vi "Execute.vi"(6 "Index [-1]":i32=-1, 7 "Composite Object":refnum<class "CConfig Object.lvclass">, 8 "error in (no error)":errorcluster, 9 "Results":string[][](array[string]), 11 "Config Query in":refnum<class "If Query.lvclass">) -> (0 "error out":errorcluster, 1 "Results":string[][](array[string]), 2 "Result":bool, 3 "Config Query out":refnum<class "If Query.lvclass">, 4 "Index":i32, 5 "Composite Object":refnum<class "CConfig Object.lvclass">)   [LabVIEW 2013, in "If Query.lvclass"]
doc: "Copyright 2018, Carya Automatisering, Wiebe Walstra."
uses:
  If Query.lvclass
  CConfig Object.lvclass
  If Query.lvclass/If Query.ctl
  CConfig Query.lvclass
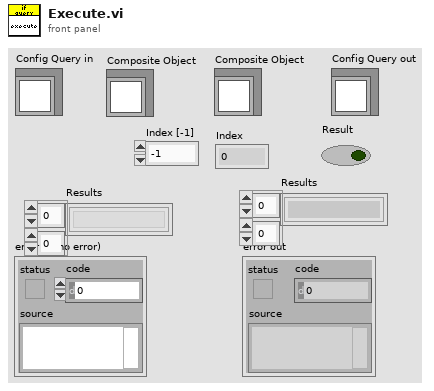
[diagram p1: front panel]
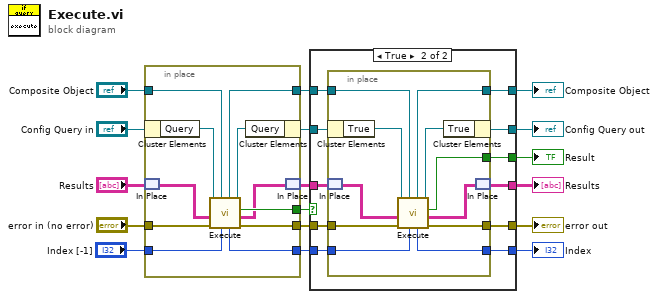
[diagram p0: block diagram]
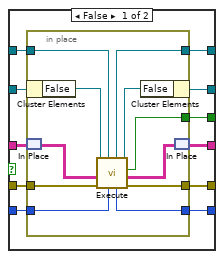
[diagram p2: hidden frame]
diagram:
  n1 = in-place {
    in-place-border: "error in (no error)" -> [w28]
    in-place-border: [w27] -> w15
    in-place-border: [w26] -> w13
    in-place-border: "Composite Object" -> [w25]
    in-place-border: "Index [-1]" -> [w24]
    in-place-border: [w23] -> w5
    in-place-border: [w20] -> w4
    n2 = in-place-cluster #1("Config Query in") -> ("Query"=w22:refnum<class "CConfig Query.lvclass">)
    n3 = in-place-match #2("Results") -> (w19:string[][])
    n4 = call-dynamic "Execute.vi"("Index [-1]"=w24, "Composite Object"=w25, "error in (no error)"=w28, "Results"=w19, "Config Query in"=w22) -> ("error out"=w27:errorcluster, "Results"=w18:string[][], "Result"=w20:bool, "Config Query out"=w21:refnum<class "CConfig Query.lvclass">, "Index"=w23:i32, "Composite Object"=w26:refnum<class "CConfig Object.lvclass">)  [unwired: 1 in]
    n5 = in-place-cluster #1("Query"=w21) -> (w6:refnum<class "If Query.lvclass">)
    n6 = in-place-match #2(w18) -> (w1:string[][])
  }
  n7 = case shown="True" w4 {
    tunnel: [w34 w56] -> w16
    tunnel: w6 -> [w35 w57]
    tunnel: w15 -> [w39 w61]
    tunnel: [w38 w60] -> w14
    tunnel: w13 -> [w37 w59]
    tunnel: [w36 w58] -> w12
    tunnel: [w33 w55] -> w11
    tunnel: [w32 w54] -> w10
    tunnel: [w29 w51] -> w3
    tunnel: w5 -> [w31 w53]
    tunnel: w1 -> [w30 w52]
    frame False {
      n8 = in-place {
        in-place-border: w39 -> [w50]
        in-place-border: [w49] -> w38
        in-place-border: w37 -> [w48]
        in-place-border: [w47] -> w36
        in-place-border: [w44] -> w33
        in-place-border: [w43] -> w32
        in-place-border: w31 -> [w42]
        n9 = in-place-cluster #3(w35) -> ("False"=w46:refnum<class "CConfig Query.lvclass">)
        n10 = in-place-match #4(w30) -> (w41:string[][])
        n11 = call-dynamic "Execute.vi"("Index [-1]"=w42, "Composite Object"=w48, "error in (no error)"=w50, "Results"=w41, "Config Query in"=w46) -> ("error out"=w49:errorcluster, "Results"=w40:string[][], "Result"=w44:bool, "Config Query out"=w45:refnum<class "CConfig Query.lvclass">, "Index"=w43:i32, "Composite Object"=w47:refnum<class "CConfig Object.lvclass">)  [unwired: 1 in]
        n12 = in-place-cluster #3("False"=w45) -> (w34:refnum<class "If Query.lvclass">)
        n13 = in-place-match #4(w40) -> (w29:string[][])
      }
    }
    frame True {
      n14 = in-place {
        in-place-border: w61 -> [w72]
        in-place-border: [w71] -> w60
        in-place-border: w59 -> [w70]
        in-place-border: [w69] -> w58
        in-place-border: [w66] -> w55
        in-place-border: w53 -> [w65]
        in-place-border: [w64] -> w54
        n15 = in-place-cluster #5(w57) -> ("True"=w68:refnum<class "CConfig Query.lvclass">)
        n16 = in-place-match #6(w52) -> (w63:string[][])
        n17 = call-dynamic "Execute.vi"("Index [-1]"=w65, "Composite Object"=w70, "error in (no error)"=w72, "Results"=w63, "Config Query in"=w68) -> ("error out"=w71:errorcluster, "Results"=w62:string[][], "Result"=w66:bool, "Config Query out"=w67:refnum<class "CConfig Query.lvclass">, "Index"=w64:i32, "Composite Object"=w69:refnum<class "CConfig Object.lvclass">)  [unwired: 1 in]
        n18 = in-place-cluster #5("True"=w67) -> (w56:refnum<class "If Query.lvclass">)
        n19 = in-place-match #6(w62) -> (w51:string[][])
      }
    }
  }
  "error out" <- w14
  "Config Query out" <- w16
  "Composite Object" <- w12
  "Result" <- w11
  "Index" <- w10
  "Results" <- w3
